vi "AG-UC2-UC8_Example.vi"() -> ()   [LabVIEW 2014]
uses:
  C:/Program Files/Newport/Piezo Motion Control/Newport AG-UC2-UC8 Applet/Samples/LabVIEW 2009/AgilisCmdLib.dll
  AgilisCmdLib.dll
panel:
  out "VE error":i32
  out "errstring":string
  out "Information":string
  in  "Instrument Key":string
  out "error out":errorcluster
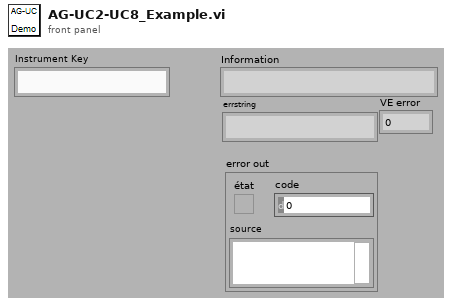
[diagram p1: front panel]
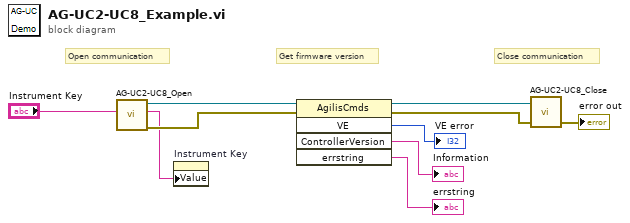
[diagram p0: block diagram]
diagram:
  # "Get firmware version"
  # "Close communication"
  # "Open communication"
  n1 = call "AG-UC2-UC8_Open.vi"("Instrument Key IN"="Instrument Key") -> ("error out"=w9:errorcluster, "Instrument Key OUT"=w1:string, "AG-UC2-UC8 Reference"=w7:refnum<k24>)  [unwired: 3 in, 1 out]
  n2 = property on="Instrument Key" class="Str"("Value"=w1) -> ()  [unwired: 2 in, 2 out]
  n3 = invoke class="AgilisCmds" method="VE"(reference=w7, error in=w9) -> (reference out=w6:refnum<k24>, error out=w8:errorcluster, "VE"=→"VE error":i32, "ControllerVersion"=→"Information":string, "errstring"=→"errstring":string)  [unwired: 3 in]
  n4 = call "AG-UC2-UC8_Close.vi"("error in (no error)"=w8, "AG-UC2-UC8 Reference"=w6) -> ("Error out"=→"error out":errorcluster)  [unwired: 2 in, 1 out]
